vi "Filter Repeatability Results.vi"(8 "error in (no error)":errorcluster, 10 "SensorID":i32, 11 "Repeatability Results":T1[](array[typedef])) -> (0 "error out":errorcluster, 3 "Repeatability Results":T1[](array[typedef]))   [LabVIEW 2026, in "Analysis.lvlib"]
uses:
  Analysis.lvlib
  Repeatability Result.ctl
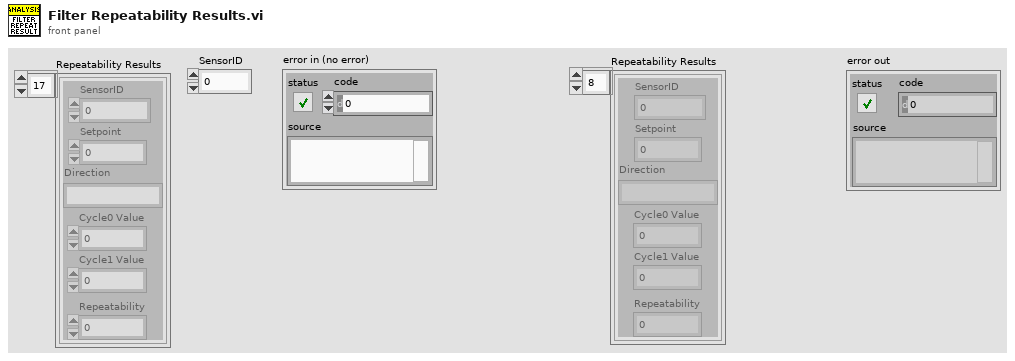
[diagram p1: front panel]
types:
  T1 = typedef "Analysis.lvlib/Repeatability Result.ctl" = cluster{"Setpoint":dbl, "Cycle0 Value":dbl, "SensorID":i32, "Cycle1 Value":dbl, "Repeatability":dbl, "Direction":string}
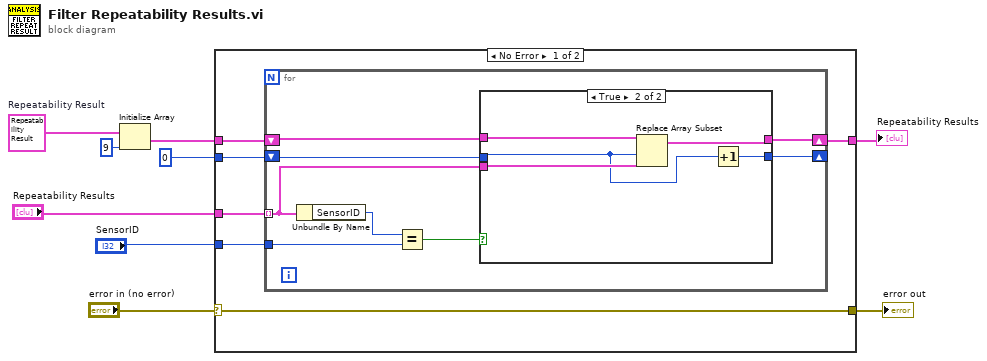
[diagram p0: block diagram]
diagram:
  w1 = T1 {"Setpoint"=99.9999494981399, "Cycle0 Value"=95.0533259725336, "SensorID"=18, "Cycle1 Value"=95.0533259725336, "Repeatability"=0.0, "Direction"="Acsending"}  # Repeatability Result
  n1 = Initialize Array(w1, 9 ("dimension size")) -> (w8:T1[])
  n2 = case shown="No Error" "error in (no error)" {
    selector: "error in (no error)" -> [w10 w32]
    tunnel: "SensorID" -> [w15 _]
    tunnel: "Repeatability Results" -> [w14 _]
    tunnel: [w13 w31] -> w2
    tunnel: w8 -> [w12 w31]
    tunnel: 0 -> [w11 _]
    tunnel: [w10 w32] -> w4
    frame No Error {
      n3 = for {
        tunnel: w14 -> [w20] mode=indexing
        tunnel: w15 -> [w22]
        shift-right: [w18] -> w13
        shift-left: w12 -> [w19]
        shift-right: [w16] -> _
        shift-left: w11 -> [w17]
        n4 = Unbundle By Name(w20) -> ("SensorID"=w23:i32)
        n5 = Equal?(x=w23, y=w22) -> (x = y?=w21:bool)
        n6 = case shown="True" w21 {
          tunnel: w20 -> [_ w28]
          tunnel: w19 -> [w25 w30]
          tunnel: [w25 w29] -> w18
          tunnel: w17 -> [w24 w27]
          tunnel: [w24 w26] -> w16
          frame False {
          }
          frame True {
            n7 = Replace Array Subset(array=w30, new element=w28, index=w27) -> (w29:T1[])
            n8 = Increment(x=w27) -> (x+1=w26:i32)
          }
        }
      }
    }
    frame Error {
    }
  }
  "error out" <- w4
  "Repeatability Results" <- w2
